vi "BTK 2 band Model.vi"(9 "V":dbl[](array[numeric])=[-0.05, -0.0499, -0.049800000000000004, -0.0497, -0.049600000000000005, -0.0495, -0.0494, -0.049300000000000004, -0.0492, -0.049100000000000005, -0.049, -0.048900000000000006, -0.0488, -0.0487, -0.048600000000000004, -0.0485, -0.048400000000000006, -0.0483, -0.0482, -0.048100000000000004, -0.048, -0.047900000000000005, -0.0478, -0.047700000000000006, -0.0476, -0.0475, -0.047400000000000005, -0.0473, -0.047200000000000006, -0.0471, -0.047, -0.046900000000000004, -0.0468, -0.046700000000000005, -0.0466, -0.0465, -0.046400000000000004, -0.0463, -0.046200000000000005, -0.0461, -0.046, -0.0459, -0.0458, -0.045700000000000005, -0.0456, -0.0455, -0.0454, -0.0453, -0.045200000000000004, -0.0451, -0.045000000000000005, -0.0449, -0.0448, -0.044700000000000004, -0.0446, -0.044500000000000005, -0.0444, -0.044300000000000006, -0.0442, -0.0441, -0.044000000000000004, -0.0439, -0.043800000000000006, -0.0437, -0.0436, -0.043500000000000004, -0.0434, -0.043300000000000005, -0.0432, -0.0431, -0.043000000000000003, -0.0429, -0.042800000000000005, -0.0427, -0.0426, -0.0425, -0.0424, -0.042300000000000004, -0.0422, -0.0421, -0.042, -0.04190000000000001, -0.041800000000000004, -0.0417, -0.0416, -0.0415, -0.041400000000000006, -0.0413, -0.0412, -0.041100000000000005, -0.041, -0.040900000000000006, -0.0408, -0.0407, -0.040600000000000004, -0.0405, -0.040400000000000005, -0.0403, -0.0402, -0.040100000000000004, -0.04, -0.039900000000000005, -0.0398, -0.0397, -0.0396, -0.0395, -0.039400000000000004, -0.0393, -0.0392, -0.0391, -0.039, -0.038900000000000004, -0.0388, -0.0387, -0.0386, -0.038500000000000006, -0.038400000000000004, -0.0383, -0.038200000000000005, -0.0381, -0.038000000000000006, -0.0379, -0.0378, -0.037700000000000004, -0.0376, -0.037500000000000006, -0.0374, -0.0373, -0.037200000000000004, -0.0371, -0.037000000000000005, -0.0369, -0.0368, -0.0367, -0.0366, -0.036500000000000005, -0.0364, -0.0363, -0.0362, -0.0361, -0.036000000000000004, -0.0359, -0.0358, -0.0357, -0.0356, -0.035500000000000004, -0.0354, -0.0353, -0.0352, -0.035100000000000006, -0.035, -0.0349, -0.034800000000000005, -0.0347, -0.034600000000000006, -0.0345, -0.0344, -0.0343, -0.0342, -0.034100000000000005, -0.034, -0.0339, -0.033800000000000004, -0.0337, -0.033600000000000005, -0.0335, -0.0334, -0.0333, -0.0332, -0.033100000000000004, -0.033, -0.0329, -0.0328, -0.03270000000000001, -0.032600000000000004, -0.0325, -0.0324, -0.0323, -0.032200000000000006, -0.032100000000000004, -0.032, -0.0319, -0.0318, -0.031700000000000006, -0.0316, -0.0315, -0.0314, -0.0313, -0.031200000000000002, -0.031100000000000003, -0.031000000000000003, -0.0309, -0.0308, -0.0307, -0.030600000000000002, -0.030500000000000003, -0.030400000000000003, -0.0303, -0.0302, -0.030100000000000002, -0.030000000000000002, -0.029900000000000003, -0.0298, -0.0297, -0.0296, -0.029500000000000002, -0.029400000000000003, -0.029300000000000003, -0.0292, -0.0291, -0.029, -0.028900000000000002, -0.028800000000000003, -0.028700000000000003, -0.0286, -0.0285, -0.0284, -0.028300000000000002, -0.028200000000000003, -0.028100000000000003, -0.028, -0.0279, -0.027800000000000002, -0.027700000000000002, -0.027600000000000003, -0.0275, -0.0274, -0.0273, -0.027200000000000002, -0.027100000000000003, -0.027000000000000003, -0.0269, -0.0268, -0.0267, -0.026600000000000002, -0.026500000000000003, -0.026400000000000003, -0.0263, -0.0262, -0.0261, -0.026000000000000002, -0.025900000000000003, -0.0258, -0.0257, -0.0256, -0.025500000000000002, -0.025400000000000002, -0.025300000000000003, -0.0252, -0.0251, -0.025, -0.024900000000000002, -0.024800000000000003, -0.024700000000000003, -0.0246, -0.0245, -0.0244, -0.024300000000000002, -0.024200000000000003, -0.0241, -0.024, -0.0239, -0.0238, -0.023700000000000002, -0.023600000000000003, -0.0235, -0.0234, -0.0233, -0.023200000000000002, -0.023100000000000002, -0.023000000000000003, -0.0229, -0.0228, -0.0227, -0.022600000000000002, -0.022500000000000003, -0.0224, -0.0223, -0.0222, -0.0221, -0.022000000000000002, -0.021900000000000003, -0.0218, -0.0217, -0.0216, -0.021500000000000002, -0.021400000000000002, -0.021300000000000003, -0.0212, -0.0211, -0.021, -0.020900000000000002, -0.020800000000000003, -0.0207, -0.0206, -0.0205, -0.0204, -0.020300000000000002, -0.020200000000000003, -0.0201, -0.02, -0.0199, -0.0198, -0.019700000000000002, -0.019600000000000003, -0.0195, -0.0194, -0.0193, -0.019200000000000002, -0.019100000000000002, -0.019000000000000003, -0.0189, -0.0188, -0.0187, -0.0186, -0.018500000000000003, -0.0184, -0.018300000000000004, -0.0182, -0.018099999999999998, -0.018000000000000002, -0.0179, -0.017800000000000003, -0.0177, -0.017600000000000005, -0.0175, -0.0174, -0.017300000000000003, -0.0172, -0.017100000000000004, -0.017, -0.0169, -0.016800000000000002, -0.0167, -0.016600000000000004, -0.0165, -0.016399999999999998, -0.016300000000000002, -0.0162, -0.016100000000000003, -0.016, -0.015900000000000004, -0.0158, -0.0157, -0.015600000000000003, -0.0155, -0.015400000000000004, -0.015300000000000001, -0.015199999999999998, -0.015100000000000002, -0.015, -0.014900000000000004, -0.0148, -0.014699999999999998, -0.014600000000000002, -0.014499999999999999, -0.014400000000000003, -0.0143, -0.014200000000000004, -0.014100000000000001, -0.013999999999999999, -0.013900000000000003, -0.0138, -0.013700000000000004, -0.013600000000000001, -0.013499999999999998, -0.013400000000000002, -0.0133, -0.013200000000000003, -0.0131, -0.012999999999999998, -0.012900000000000002, -0.012799999999999999, -0.012700000000000003, -0.0126, -0.012500000000000004, -0.012400000000000001, -0.012299999999999998, -0.012200000000000003, -0.0121, -0.012000000000000004, -0.0119, -0.011799999999999998, -0.011700000000000002, -0.0116, -0.011500000000000003, -0.0114, -0.011299999999999998, -0.011200000000000002, -0.011099999999999999, -0.011000000000000003, -0.0109, -0.010800000000000004, -0.010700000000000001, -0.010599999999999998, -0.010500000000000002, -0.0104, -0.010300000000000004, -0.0102, -0.010099999999999998, -0.010000000000000002, -0.009899999999999999, -0.009800000000000003, -0.0097, -0.009599999999999997, -0.009500000000000001, -0.009399999999999999, -0.009300000000000003, -0.0092, -0.009100000000000004, -0.009000000000000001, -0.008899999999999998, -0.008800000000000002, -0.0087, -0.008600000000000003, -0.0085, -0.008399999999999998, -0.008300000000000002, -0.008199999999999999, -0.008100000000000003, -0.008, -0.007899999999999997, -0.007800000000000001, -0.0076999999999999985, -0.007600000000000003, -0.0075, -0.007400000000000004, -0.007300000000000001, -0.007199999999999998, -0.007100000000000002, -0.006999999999999999, -0.006900000000000003, -0.0068000000000000005, -0.006699999999999998, -0.006600000000000002, -0.006499999999999999, -0.006400000000000003, -0.0063, -0.006200000000000004, -0.006100000000000001, -0.005999999999999998, -0.0059000000000000025, -0.0058, -0.005700000000000004, -0.005600000000000001, -0.005499999999999998, -0.005400000000000002, -0.005299999999999999, -0.005200000000000003, -0.0051, -0.0049999999999999975, -0.004900000000000002, -0.004799999999999999, -0.004700000000000003, -0.0046, -0.004500000000000004, -0.004400000000000001, -0.004299999999999998, -0.004200000000000002, -0.0040999999999999995, -0.0040000000000000036, -0.0039000000000000007, -0.003799999999999998, -0.003700000000000002, -0.003599999999999999, -0.003500000000000003, -0.0034000000000000002, -0.0032999999999999974, -0.0032000000000000015, -0.0030999999999999986, -0.0030000000000000027, -0.0029, -0.002800000000000004, -0.002700000000000001, -0.002599999999999998, -0.0025000000000000022, -0.0023999999999999994, -0.0023000000000000034, -0.0022000000000000006, -0.0020999999999999977, -0.0020000000000000018, -0.001899999999999999, -0.001800000000000003, -0.0017000000000000001, -0.0015999999999999973, -0.0015000000000000013, -0.0013999999999999985, -0.0013000000000000025, -0.0011999999999999997, -0.0011000000000000038, -0.0010000000000000009, -0.000899999999999998, -0.0008000000000000021, -0.0006999999999999992, -0.0006000000000000033, -0.0005000000000000004, -0.0003999999999999976, -0.00030000000000000165, -0.0001999999999999988, -0.00010000000000000286, 0.0, 0.00010000000000000286, 0.0001999999999999988, 0.00030000000000000165, 0.0003999999999999976, 0.0005000000000000004, 0.0005999999999999964, 0.0006999999999999992, 0.0008000000000000021, 0.000899999999999998, 0.0010000000000000009, 0.0010999999999999968, 0.0011999999999999997, 0.0013000000000000025, 0.0013999999999999985, 0.0015000000000000013, 0.0015999999999999973, 0.0017000000000000001, 0.001800000000000003, 0.001899999999999999, 0.0020000000000000018, 0.0020999999999999977, 0.0022000000000000006, 0.0022999999999999965, 0.0023999999999999994, 0.0025000000000000022, 0.002599999999999998, 0.002700000000000001, 0.002799999999999997, 0.0029, 0.0030000000000000027, 0.0030999999999999986, 0.0032000000000000015, 0.0032999999999999974, 0.0034000000000000002, 0.003500000000000003, 0.003599999999999999, 0.003700000000000002, 0.003799999999999998, 0.0039000000000000007, 0.003999999999999997, 0.0040999999999999995, 0.004200000000000002, 0.004299999999999998, 0.004400000000000001, 0.004499999999999997, 0.0046, 0.004700000000000003, 0.004799999999999999, 0.004900000000000002, 0.0049999999999999975, 0.0051, 0.005200000000000003, 0.005299999999999999, 0.005400000000000002, 0.005499999999999998, 0.005600000000000001, 0.005699999999999997, 0.0058, 0.0059000000000000025, 0.005999999999999998, 0.006100000000000001, 0.006199999999999997, 0.0063, 0.006400000000000003, 0.006499999999999999, 0.006600000000000002, 0.006699999999999998, 0.0068000000000000005, 0.006900000000000003, 0.006999999999999999, 0.007100000000000002, 0.007199999999999998, 0.007300000000000001, 0.007399999999999997, 0.0075, 0.007600000000000003, 0.0076999999999999985, 0.007800000000000001, 0.007899999999999997, 0.008, 0.008100000000000003, 0.008199999999999999, 0.008300000000000002, 0.008399999999999998, 0.0085, 0.008600000000000003, 0.0087, 0.008800000000000002, 0.008899999999999998, 0.009000000000000001, 0.009099999999999997, 0.0092, 0.009300000000000003, 0.009399999999999999, 0.009500000000000001, 0.009599999999999997, 0.0097, 0.009800000000000003, 0.009899999999999999, 0.010000000000000002, 0.010099999999999998, 0.0102, 0.010299999999999997, 0.0104, 0.010500000000000002, 0.010599999999999998, 0.010700000000000001, 0.010799999999999997, 0.0109, 0.011000000000000003, 0.011099999999999999, 0.011200000000000002, 0.011299999999999998, 0.0114, 0.011500000000000003, 0.0116, 0.011700000000000002, 0.011799999999999998, 0.0119, 0.011999999999999997, 0.0121, 0.012200000000000003, 0.012299999999999998, 0.012400000000000001, 0.012499999999999997, 0.0126, 0.012700000000000003, 0.012800000000000006, 0.012899999999999995, 0.012999999999999998, 0.0131, 0.013200000000000003, 0.013300000000000006, 0.013399999999999995, 0.013499999999999998, 0.013600000000000001, 0.013700000000000004, 0.013800000000000007, 0.013899999999999996, 0.013999999999999999, 0.014100000000000001, 0.014200000000000004, 0.014300000000000007, 0.014399999999999996, 0.014499999999999999, 0.014600000000000002, 0.014700000000000005, 0.014799999999999994, 0.014899999999999997, 0.015, 0.015100000000000002, 0.015200000000000005, 0.015299999999999994, 0.015399999999999997, 0.0155, 0.015600000000000003, 0.015700000000000006, 0.015799999999999995, 0.015899999999999997, 0.016, 0.016100000000000003, 0.016200000000000006, 0.016299999999999995, 0.016399999999999998, 0.0165, 0.016600000000000004, 0.016700000000000007, 0.016799999999999995, 0.0169, 0.017, 0.017100000000000004, 0.017200000000000007, 0.017299999999999996, 0.0174, 0.0175, 0.017600000000000005, 0.017700000000000007, 0.017799999999999996, 0.0179, 0.018000000000000002, 0.018100000000000005, 0.018199999999999994, 0.018299999999999997, 0.0184, 0.018500000000000003, 0.018600000000000005, 0.018699999999999994, 0.018799999999999997, 0.0189, 0.019000000000000003, 0.019100000000000006, 0.019199999999999995, 0.019299999999999998, 0.0194, 0.019500000000000003, 0.019600000000000006, 0.019699999999999995, 0.019799999999999998, 0.0199, 0.020000000000000004, 0.020100000000000007, 0.020199999999999996, 0.0203, 0.0204, 0.020500000000000004, 0.020600000000000007, 0.020699999999999996, 0.0208, 0.020900000000000002, 0.021000000000000005, 0.021099999999999994, 0.021199999999999997, 0.0213, 0.021400000000000002, 0.021500000000000005, 0.021599999999999994, 0.021699999999999997, 0.0218, 0.021900000000000003, 0.022000000000000006, 0.022099999999999995, 0.022199999999999998, 0.0223, 0.022400000000000003, 0.022500000000000006, 0.022599999999999995, 0.022699999999999998, 0.0228, 0.022900000000000004, 0.023000000000000007, 0.023099999999999996, 0.0232, 0.0233, 0.023400000000000004, 0.023500000000000007, 0.023599999999999996, 0.0237, 0.0238, 0.023900000000000005, 0.024000000000000007, 0.024099999999999996, 0.0242, 0.024300000000000002, 0.024400000000000005, 0.024499999999999994, 0.024599999999999997, 0.0247, 0.024800000000000003, 0.024900000000000005, 0.024999999999999994, 0.025099999999999997, 0.0252, 0.025300000000000003, 0.025400000000000006, 0.025499999999999995, 0.025599999999999998, 0.0257, 0.025800000000000003, 0.025900000000000006, 0.025999999999999995, 0.026099999999999998, 0.0262, 0.026300000000000004, 0.026400000000000007, 0.026499999999999996, 0.0266, 0.0267, 0.026800000000000004, 0.026900000000000007, 0.026999999999999996, 0.0271, 0.027200000000000002, 0.027300000000000005, 0.027400000000000008, 0.027499999999999997, 0.0276, 0.027700000000000002, 0.027800000000000005, 0.027899999999999994, 0.027999999999999997, 0.0281, 0.028200000000000003, 0.028300000000000006, 0.028399999999999995, 0.028499999999999998, 0.0286, 0.028700000000000003, 0.028800000000000006, 0.028899999999999995, 0.028999999999999998, 0.0291, 0.029200000000000004, 0.029300000000000007, 0.029399999999999996, 0.0295, 0.0296, 0.029700000000000004, 0.029800000000000007, 0.029899999999999996, 0.03, 0.030100000000000002, 0.030200000000000005, 0.030300000000000007, 0.030399999999999996, 0.0305, 0.030600000000000002, 0.030700000000000005, 0.030800000000000008, 0.030899999999999997, 0.031, 0.031100000000000003, 0.031200000000000006, 0.031299999999999994, 0.0314, 0.0315, 0.0316, 0.031700000000000006, 0.031799999999999995, 0.0319, 0.032, 0.032100000000000004, 0.032200000000000006, 0.032299999999999995, 0.0324, 0.0325, 0.032600000000000004, 0.03270000000000001, 0.032799999999999996, 0.0329, 0.033, 0.033100000000000004, 0.03320000000000001, 0.033299999999999996, 0.0334, 0.0335, 0.033600000000000005, 0.03370000000000001, 0.0338, 0.0339, 0.034, 0.034100000000000005, 0.03420000000000001, 0.0343, 0.0344, 0.0345, 0.034600000000000006, 0.034699999999999995, 0.0348, 0.0349, 0.035, 0.035100000000000006, 0.035199999999999995, 0.0353, 0.0354, 0.035500000000000004, 0.03560000000000001, 0.035699999999999996, 0.0358, 0.0359, 0.036000000000000004, 0.03610000000000001, 0.036199999999999996, 0.0363, 0.0364, 0.036500000000000005, 0.03660000000000001, 0.036699999999999997, 0.0368, 0.0369, 0.037000000000000005, 0.03710000000000001, 0.0372, 0.0373, 0.0374, 0.037500000000000006, 0.037599999999999995, 0.0377, 0.0378, 0.0379, 0.038000000000000006, 0.038099999999999995, 0.0382, 0.0383, 0.038400000000000004, 0.038500000000000006, 0.038599999999999995, 0.0387, 0.0388, 0.038900000000000004, 0.03900000000000001, 0.039099999999999996, 0.0392, 0.0393, 0.039400000000000004, 0.03950000000000001, 0.039599999999999996, 0.0397, 0.0398, 0.039900000000000005, 0.04000000000000001, 0.0401, 0.0402, 0.0403, 0.040400000000000005, 0.04050000000000001, 0.0406, 0.0407, 0.0408, 0.040900000000000006, 0.040999999999999995, 0.0411, 0.0412, 0.0413, 0.041400000000000006, 0.041499999999999995, 0.0416, 0.0417, 0.041800000000000004, 0.04190000000000001, 0.041999999999999996, 0.0421, 0.0422, 0.042300000000000004, 0.04240000000000001, 0.042499999999999996, 0.0426, 0.0427, 0.042800000000000005, 0.04290000000000001, 0.043, 0.0431, 0.0432, 0.043300000000000005, 0.04340000000000001, 0.0435, 0.0436, 0.0437, 0.043800000000000006, 0.04390000000000001, 0.044, 0.0441, 0.0442, 0.044300000000000006, 0.044399999999999995, 0.0445, 0.0446, 0.044700000000000004, 0.044800000000000006, 0.044899999999999995, 0.045, 0.0451, 0.045200000000000004, 0.04530000000000001, 0.045399999999999996, 0.0455, 0.0456, 0.045700000000000005, 0.04580000000000001, 0.045899999999999996, 0.046, 0.0461, 0.046200000000000005, 0.04630000000000001, 0.0464, 0.0465, 0.0466, 0.046700000000000005, 0.04680000000000001, 0.0469, 0.047, 0.0471, 0.047200000000000006, 0.04730000000000001, 0.0474, 0.0475, 0.0476, 0.047700000000000006, 0.047799999999999995, 0.0479, 0.048, 0.048100000000000004, 0.04820000000000001, 0.048299999999999996, 0.0484, 0.0485, 0.048600000000000004, 0.04870000000000001, 0.048799999999999996, 0.0489, 0.049, 0.049100000000000005, 0.04920000000000001, 0.0493, 0.0494, 0.0495, 0.049600000000000005, 0.04970000000000001, 0.0498, 0.0499, 0.05], 10 "Parameters":T1={"Delta 1"=0.00075, "Delta 2"=0.001501, "Gama"=0.0, "Z"=0.0, "P"=0.0, "T"=1.5, "Integration range"=1.0, "Resolution"=0.0001} {"Delta 1" step=0.001 format="%#_6peV"; "Resolution" format="%#_6peV"; "Integration range" format="%#_6peV"; "T" format="%#_6pK"; "Delta 2" step=0.001 format="%#_6peV"; "Gama" step=0.001 format="%#_6peV"}) -> (2 "Conductivity":dbl[](array[numeric]))   [LabVIEW 2021]
uses:
  Parameters.ctl
panel:
  out "Waveform Graph":dbl[][](graph)
  out "XY Graph":cluster{dbl[], dbl[]}(graph)
  in  "Normalize":bool
  out "I-V":cluster{"Steps":dbl[], "dX/dt":dbl[]}(graph)
  out "f(E-eV)-f(E)":cluster{"Steps":dbl[], "dX/dt":dbl[]}(graph)
  out "Z":cluster{"Steps":dbl[], "dX/dt":dbl[]}(graph)
  out "dIdV":cluster{"Steps":dbl[], "dX/dt":dbl[]}(graph)
  # "<="
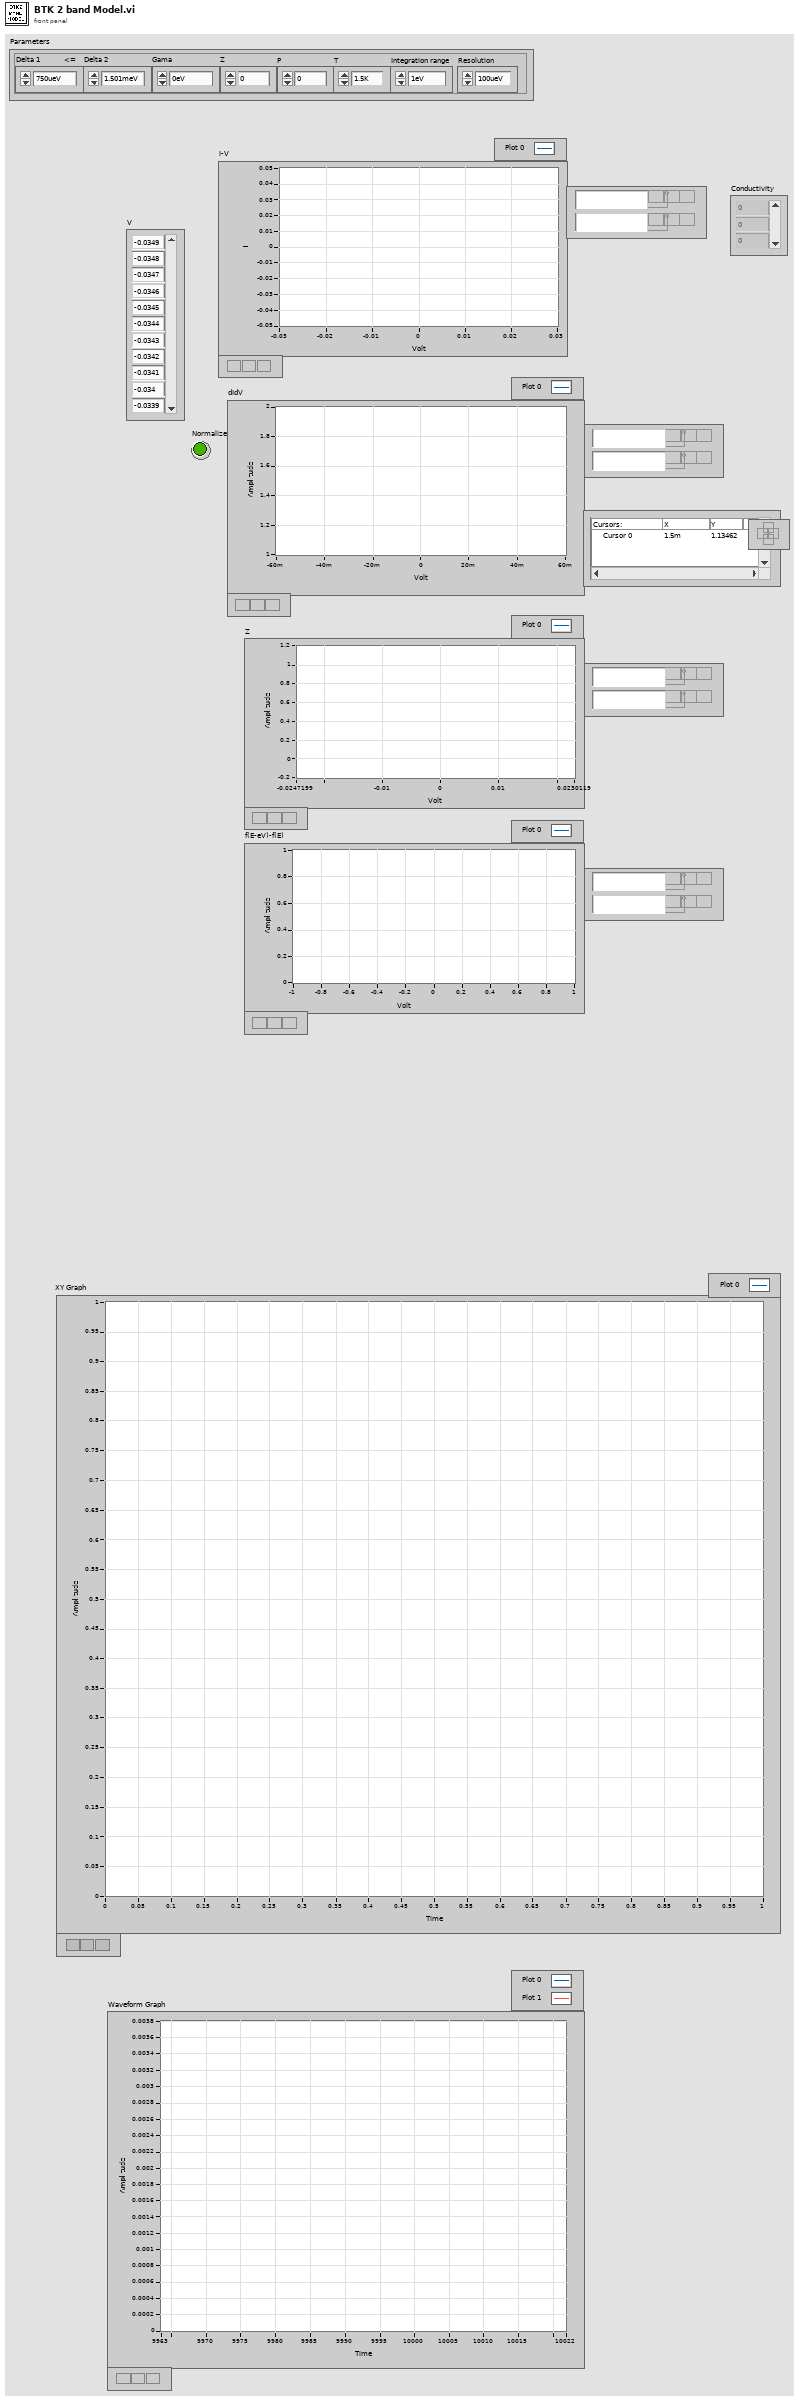
[diagram p1: front panel]
types:
  T1 = typedef "Parameters.ctl" = cluster{"Delta 1":dbl, "Delta 2":dbl, "Gama":dbl, "Z":dbl, "P":dbl, "T":dbl, "Integration range":dbl, "Resolution":dbl}
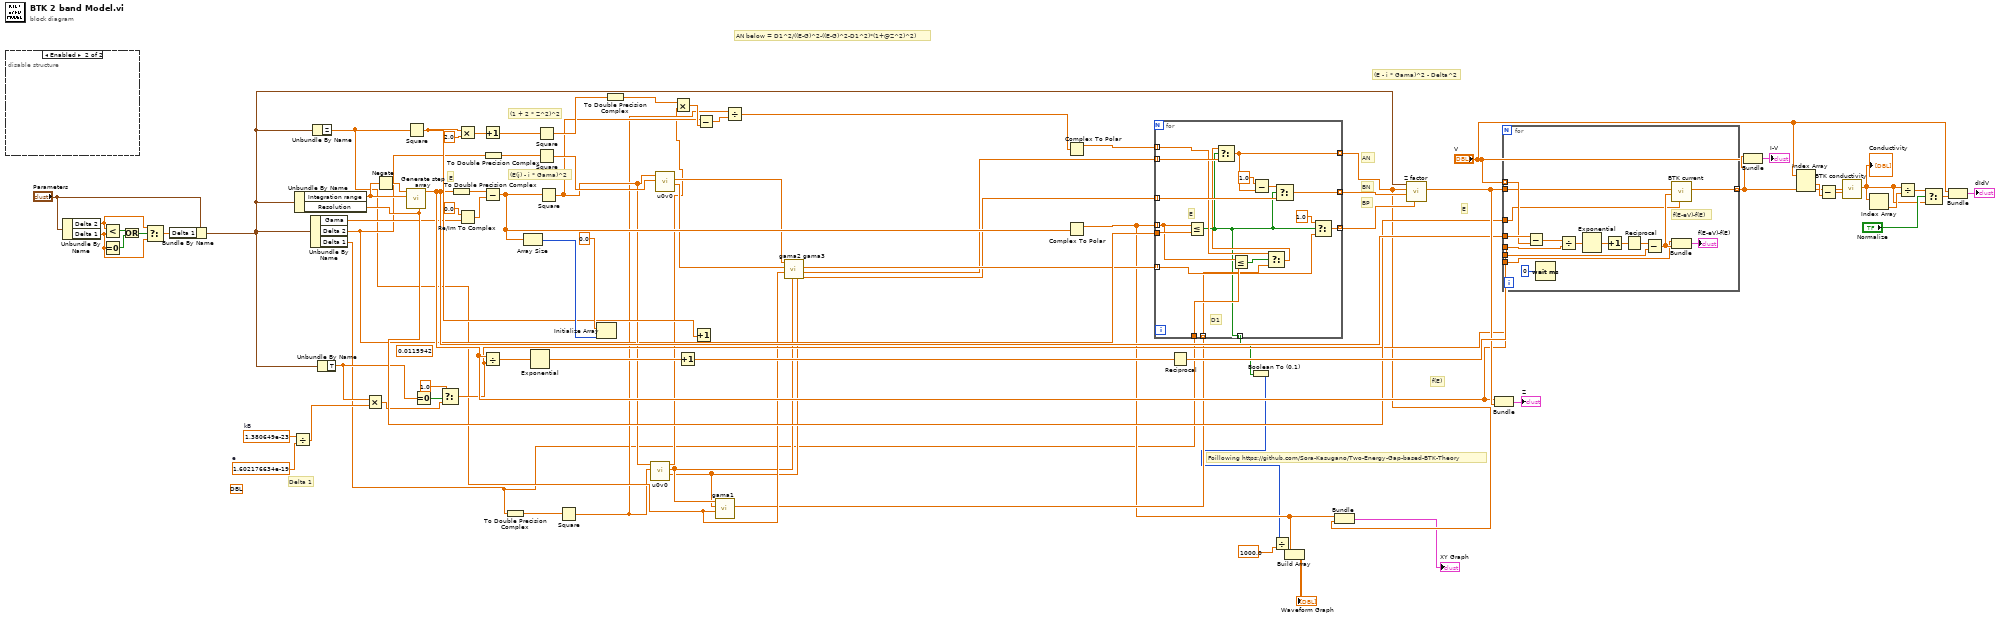
[diagram p0: block diagram]
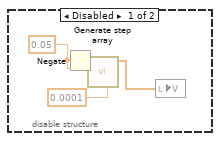
[diagram p2: hidden frame]
diagram:
  w52 = 1.602176634e-19  # e
  (unwired) ext[unit] 1.602176634e-19
  w53 = 1.380649e-23  # kB
  (unwired) 0.0115942
  # "Delta 1"
  # "f(E)"
  # "E"
  # "BP"
  # "BN"
  # "AN"
  # "Foillowing https://github.com/Sora-Kasugano/Two-Energy-Gap-based-BTK-Theory"
  # "AN below = D1^2/((E-G)^2-((E-G)^2-D1^2)*(1+@Z^2)^2)"
  # "(E(j) - i * Gama)^2"
  # "(E - i * Gama)^2 - Delta^2"
  # "(1 + 2 * Z^2)^2"
  # "E"
  n1 = disable-structure shown="Enabled" {
    frame Disabled {
      w85 = 0.05 ("Start")
      n2 = Negate(x=w85) -> (-x=w84:dbl)
      n3 = call "Generate step array.vi"("Step"=0.0001, "End"=w85, "Start"=w84) -> ("Steps"=w86:dbl[])  [unwired: 8 in]
      n4 = local write "V"(w86) -> ()
    }
    frame Enabled {
    }
  }
  n5 = Unbundle By Name("Parameters") -> ("Delta 2"=w4:dbl, "Delta 1"=w3:dbl)
  n6 = Less?(x=w4, y=w3) -> (x < y?=w8:bool)
  n7 = Equal To 0?(x=w3) -> (x = 0?=w7:bool)
  n8 = Or(x=w8, y=w7) -> (x .or. y?=w5:bool)
  n9 = Select(t=w4, s=w5, f=w3) -> (s? t:f=w2:dbl)
  n10 = Bundle By Name(cluster="Parameters", "Delta 1"=w2) -> (w1:T1)
  n11 = Divide(x=w53, y=w52) -> (x/y=w41:dbl)
  n12 = Unbundle By Name(w1) -> ("Integration range"=w34:dbl, "Resolution"=w48:dbl)
  n13 = Unbundle By Name(w1) -> ("Gama"=w30:dbl, "Delta 2"=w29:dbl, "Delta 1"=w9:dbl)
  n14 = Unbundle By Name(w1) -> ("Z"=w28:dbl)
  n15 = Unbundle By Name(w1) -> ("T"=w40:dbl)
  n16 = Multiply(x=w40, y=w41) -> (x*y=w42:dbl)
  n17 = Negate(x=w34) -> (-x=w33:dbl)
  n18 = call "Generate step array.vi"("Step"=w48, "End"=w34, "Start"=w33) -> ("Steps"=w55:dbl[])  [unwired: 8 in]
  n19 = Square(x=w28) -> (x^2=w66:dbl)
  n20 = Equal To 0?(x=w40) -> (x = 0?=w45:bool)
  n21 = Select(t=1.0, s=w45, f=w42) -> (s? t:f=w43:dbl)
  n22 = To Double Precision Complex(1:w55) -> (0:w81:cdb[])
  n23 = Multiply(x=w66, y=2.0) -> (x*y=w75:dbl)
  n24 = Re/Im To Complex(1:w30, 2:0.0) -> (0:w80:cdb)
  n25 = Increment(x=w75) -> (x+1=w74:dbl)
  n26 = Subtract(x=w81, y=w80) -> (x-y=w67:cdb[])
  n27 = Divide(x=w55, y=w43) -> (x/y=w64:dbl[])
  n28 = To Double Precision Complex(1:w29) -> (0:w79:cdb)
  n29 = To Double Precision Complex(1:w9) -> (0:w32:cdb)
  n30 = Array Size(array=w67) -> (size(s)=w77:i32)
  n31 = Exponential(1:w64) -> (0:w63:dbl[])
  n32 = Square(x=w74) -> (x^2=w73:dbl)
  n33 = Square(x=w79) -> (x^2=w69:cdb)
  n34 = Square(x=w67) -> (x^2=w31:cdb[])
  n35 = Square(x=w32) -> (x^2=w24:cdb)
  n36 = Initialize Array(0.0, w77) -> ()  [unwired: 1 out]
  n37 = To Double Precision Complex(1:w73) -> (0:w72:cdb)
  n38 = call "u0v0.vi"("Delta^2"=w24, "(E-iG)^2"=w31) -> ("v0^2"=w20:dbl[], "u0^2"=w21:dbl[], "(E - i * G)^2 - Delta^2"=w18:cdb[])  [unwired: 7 in]
  n39 = call "u0v0.vi"("Delta^2"=w69, "(E-iG)^2"=w31) -> ("v0^2"=w26:dbl[], "u0^2"=w27:dbl[])  [unwired: 7 in, 1 out]
  n40 = Multiply(x=w72, y=w18) -> (x*y=w71:cdb[])
  n41 = Increment(x=w63) -> (x+1=w62:dbl[])
  n42 = Increment(x=w66) -> ()  [unwired: 1 out]
  n43 = Subtract(x=w31, y=w71) -> (x-y=w70:cdb[])
  n44 = call "gama1.vi"("Z"=w28, "v0^2"=w20, "u0^2"=w21) -> ("Au middle"=w23:dbl[])  [unwired: 6 in, 2 out]
  n45 = Divide(x=w24, y=w70) -> (x/y=w68:cdb[])
  n46 = call "gama2 gama3.vi"("v01^2"=w20, "u01^2"=w21, "Z"=w28, "v02^2"=w26, "u02^2"=w27) -> ("Bu above"=w19:dbl[], "Au above"=w22:dbl[], "Bp above"=w25:dbl[])  [unwired: 3 in, 1 out]
  n47 = Complex To Polar(r * e^(i*theta)=w68) -> (r=w65:dbl[])  [unwired: 1 out]
  n48 = Complex To Polar(r * e^(i*theta)=w67) -> (r=w15:dbl[])  [unwired: 1 out]
  n49 = for {
    tunnel: w15 -> [w94] mode=indexing
    tunnel: w29 -> [w100]
    tunnel: w65 -> [w90] mode=indexing
    tunnel: w19 -> [w99] mode=indexing
    tunnel: w22 -> [w98] mode=indexing
    tunnel: [w97] -> w17 mode=indexing
    tunnel: [w96] -> w60 mode=indexing
    tunnel: [w95] -> w59 mode=indexing
    tunnel: w9 -> [w93]
    tunnel: w25 -> [w92] mode=indexing
    tunnel: w23 -> [w88] mode=indexing
    tunnel: [w87] -> w14 mode=indexing
    # "D1"
    # "E"
    n50 = Less Or Equal?(x=w94, y=w100) -> (x <= y?=w87:bool)
    n51 = Less Or Equal?(x=w94, y=w93) -> (x <= y?=w91:bool)
    n52 = Select(t=w90, s=w91, f=w88) -> (s? t:f=w89:dbl)
    n53 = Select(t=w89, s=w87, f=w98) -> (s? t:f=w97:dbl)
    n54 = Subtract(x=1.0, y=w97) -> (x-y=w103:dbl)
    n55 = Select(t=w103, s=w87, f=w99) -> (s? t:f=w96:dbl)
    n56 = Select(t=1.0, s=w87, f=w92) -> (s? t:f=w95:dbl)
  }
  n57 = Reciprocal(x=w62) -> (1/x=w61:dbl[])
  n58 = Boolean To (0,1)(Boolean=w14) -> (0, 1=w12:i16[])
  n59 = Divide(x=w12, y=1000.0) -> (x/y=w11:dbl[])
  n60 = Build Array(w15, w11) -> (→"Waveform Graph":dbl[][])
  n61 = Bundle(w15, w17) -> (→"XY Graph":cluster{dbl[], dbl[]})  [unwired: 1 in]
  n62 = call "Z factor.vi"("BP"=w59, "BN"=w60, "AN"=w17, "Parameters"=w1) -> ("z factor"=w57:dbl[])  [unwired: 7 in]
  n63 = Bundle("Steps"=w55, "z factor"=w57) -> (→"Z":cluster{"Steps":dbl[], "z factor":dbl[]})  [unwired: 1 in]
  n64 = for {
    tunnel: "V" -> [w118] mode=indexing
    tunnel: w55 -> [w119]
    tunnel: w43 -> [w115]
    tunnel: w61 -> [w113]
    tunnel: w57 -> [w110]
    tunnel: [w109] -> w47 mode=indexing
    tunnel: w55 -> [w105]
    tunnel: w48 -> [w104]
    # "f(E-eV)-f(E)"
    n65 = Subtract(x=w119, y=w118) -> (x-y=w117:dbl[])
    n66 = Wait (ms)(milliseconds to wait=u32 0) -> ()  [unwired: 1 out]
    n67 = Divide(x=w117, y=w115) -> (x/y=w116:dbl[])
    n68 = Exponential(1:w116) -> (0:w114:dbl[])
    n69 = Increment(x=w114) -> (x+1=w112:dbl[])
    n70 = Reciprocal(x=w112) -> (1/x=w111:dbl[])
    n71 = Subtract(x=w111, y=w113) -> (x-y=w108:dbl[])
    n72 = call "BTK current.vi"("dx"=w104, "f factor"=w108, "z factor"=w110) -> ("I current"=w109:dbl)  [unwired: 8 in]
    n73 = Bundle("Steps"=w105, w108) -> (→"f(E-eV)-f(E)":cluster{"Steps":dbl[], dbl[]})  [unwired: 1 in]
  }
  n74 = Bundle(w47, "V"="V") -> (→"I-V":cluster{dbl[], "V":dbl[]})  [unwired: 1 in]
  n75 = Index Array(array="V") -> (element #1=w51:dbl, element #2=w50:dbl)  [unwired: 2 in]
  n76 = Subtract(x=w50, y=w51) -> (x-y=w49:dbl)
  n77 = call "BTK conductivity.vi"("dx"=w49, "Current"=w47) -> ("Conductivity"=w36:dbl[])  [unwired: 8 in, 1 out]
  "Conductivity" <- w36
  n78 = Index Array(array=w36) -> (element=w39:dbl)  [unwired: 1 in]
  n79 = Divide(x=w36, y=w39) -> (x/y=w38:dbl[])
  n80 = Select(t=w38, s="Normalize", f=w36) -> (s? t:f=w35:dbl[])
  n81 = Bundle("V"="V", "Conductivity"=w35) -> (→"dIdV":cluster{"V":dbl[], "Conductivity":dbl[]})  [unwired: 1 in]
